vi "Cuboid preprocessing.vi"(1 "Cuboid properties in":T1={"Vertices (x, y)"=[[0.0, 0.0, 0.0], [1.0, 0.0, 0.0], [1.0, 1.0, 0.0], [0.0, 1.0, 0.0]], "Zmin"=0.0, "Zmax"=1.0, "Centroid (x, y)"=[0.0, 0.0, 0.0], "Radius"=0.0, "Edge normals (x, y)"=[[0.0, 0.0, 0.0], [0.0, 0.0, 0.0], [0.0, 0.0, 0.0], [0.0, 0.0, 0.0]], "Edge vectors (x, y)"=[[0.0, 0.0], [0.0, 0.0], [0.0, 0.0], [0.0, 0.0]]}) -> (0 "Cuboid properties out":T1={"Vertices (x, y)"=[[0.0, 0.0, 0.0], [1.0, 0.0, 0.0], [1.0, 1.0, 0.0], [0.0, 1.0, 0.0]], "Zmin"=0.0, "Zmax"=1.0, "Centroid (x, y)"=[0.5, 0.5, 0.0], "Radius"=0.7071067811865476, "Edge normals (x, y)"=[[0.0, -1.0, 0.0], [1.0, 0.0, 0.0], [0.0, 1.0, 0.0], [-1.0, 0.0, 0.0]], "Edge vectors (x, y)"=[[1.0, 0.0, 0.0], [0.0, 1.0, 0.0], [-1.0, 0.0, 0.0], [0.0, -1.0, 0.0]]})   [LabVIEW 2013]
uses:
  Cuboids sub vis/Cuboid properties.ctl
  <vilib>/Analysis/_algsub.llb/Real Vector Norm.vi
  <vilib>/Analysis/baseanly.llb/Unit Vector (DBL).vi
  <vilib>/Analysis/baseanly.llb/Real Dot Product.vi
  <vilib>/Analysis/NI_AALBase.lvlib
  <vilib>/Analysis/NI_AALPro.lvlib
panel:
  # "PN 30/08/2014"
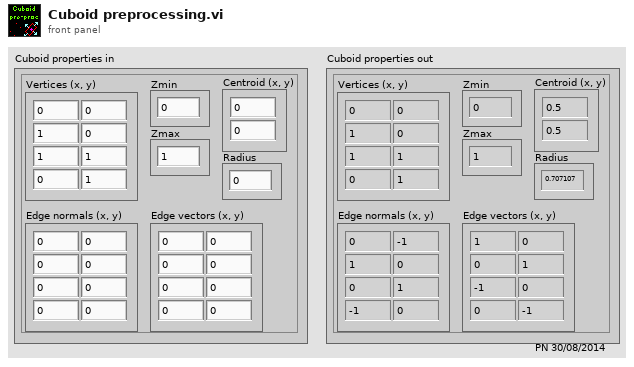
[diagram p1: front panel]
types:
  T1 = typedef "Cuboid properties.ctl" = cluster{"Vertices (x, y)":dbl[][], "Zmin":dbl, "Zmax":dbl, "Centroid (x, y)":dbl[], "Radius":dbl, "Edge normals (x, y)":dbl[][], "Edge vectors (x, y)":dbl[][]}
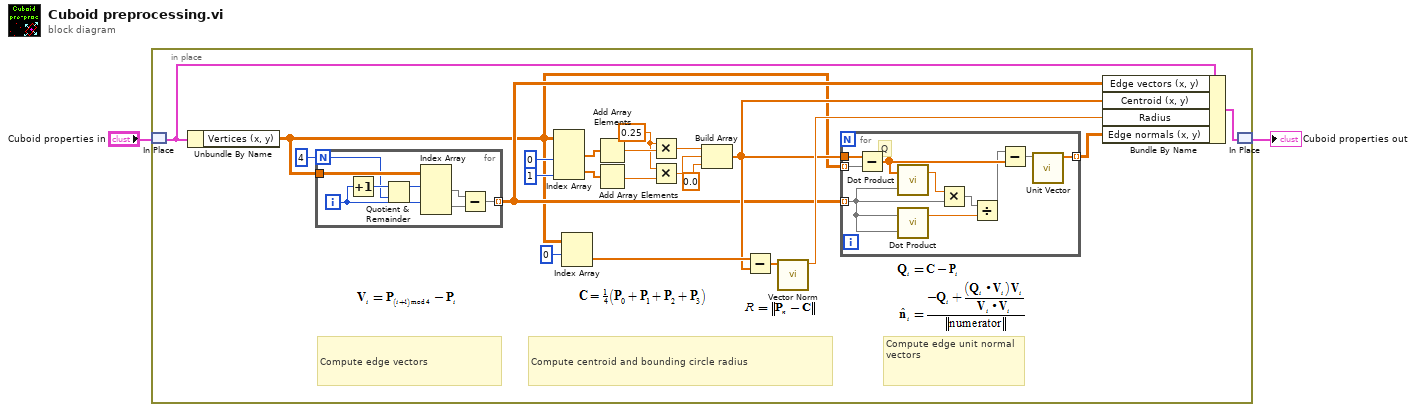
[diagram p0: block diagram]
diagram:
  n1 = in-place {
    w17 = 0.25 ("x")
    # "Compute edge unit normal vectors"
    # "Compute centroid and bounding circle radius"
    # "Compute edge vectors"
    n2 = in-place-match #1("Cuboid properties in") -> (w9:T1)
    n3 = Unbundle By Name(w9) -> ("Vertices (x, y)"=w3:dbl[][])
    n4 = for {
      N: 4 -> [w25]
      tunnel: [w27] -> w6 mode=indexing
      tunnel: w3 -> [w31]
      i -> [w30]
      n5 = Increment(x=w30) -> (x+1=w26:i32)
      n6 = Quotient & Remainder(x=w26, y=w25) -> (x-y*floor(x/y)=w24:i32)  [unwired: 1 out]
      n7 = Index Array(array=w31, index (row) #1=w24, index (row) #2=w30) -> (element #1=w29:dbl[], element #2=w28:dbl[])  [unwired: 2 in]
      n8 = Subtract(x=w29, y=w28) -> (x-y=w27:dbl[])
    }
    n9 = Index Array(array=w3, index (col) #1=0 ("disabled index (col)"), index (col) #2=1 ("index (col)")) -> (element #1=w21:dbl[], element #2=w20:dbl[])  [unwired: 2 in]
    n10 = Index Array(array=w3, index (row)=0) -> (element=w12:dbl[])  [unwired: 1 in]
    n11 = Add Array Elements(numeric array=w21) -> (sum=w19:dbl)
    n12 = Add Array Elements(numeric array=w20) -> (sum=w18:dbl)
    n13 = Multiply(x=w17, y=w19) -> (x*y=w16:dbl)
    n14 = Multiply(x=w17, y=w18) -> (x*y=w15:dbl)
    n15 = Build Array(w16, w15, 0.0 ("element")) -> (w8:dbl[])
    n16 = Subtract(x=w12, y=w8) -> (x-y=w11:dbl[])
    n17 = call-poly <vilib>:"Vector Norm.vi"("Input Vector"=w11) -> ("norm"=w10:dbl)  [unwired: 9 in, 1 out]
    n18 = for {
      tunnel: [w41] -> w7 mode=indexing
      tunnel: w6 -> [w36] mode=indexing
      tunnel: w8 -> [w40]
      tunnel: w3 -> [w39] mode=indexing
      # "Q"
      n19 = Subtract(x=w40, y=w39) -> (x-y=w38:dbl[])
      n20 = call-poly <vilib>:"Dot Product.vi"("Y Vector"=w36, "X Vector"=w38) -> ("X * Y"=w37:dbl)  [unwired: 1 out]
      n21 = call-poly <vilib>:"Dot Product.vi"("Y Vector"=w36, "X Vector"=w36) -> ("X * Y"=w35:dbl)  [unwired: 1 out]
      n22 = Multiply(x=w37, y=w36) -> (x*y=w34:dbl[])
      n23 = Divide(x=w34, y=w35) -> (x/y=w33:dbl[])
      n24 = Subtract(x=w33, y=w38) -> (x-y=w32:dbl[])
      n25 = call-poly <vilib>:"Unit Vector.vi"("Input Vector"=w32) -> ("Unit Vector"=w41:dbl[])  [unwired: 8 in, 2 out]
    }
    n26 = Bundle By Name(cluster=w9, "Edge vectors (x, y)"=w6, "Centroid (x, y)"=w8, "Radius"=w10, "Edge normals (x, y)"=w7) -> (w5:T1)
    n27 = in-place-match #1(w5) -> (→"Cuboid properties out":T1)
  }
